vi "Render.vi"(8 "error in (no error)":errorcluster, 9 "IDrawable":refnum<class "IDrawable.lvclass">, 10 "2D Picture in":picture, 11 "2DPictureControl in":refnum<class "2DPictureControl.lvclass">) -> (0 "error out":errorcluster, 2 "2D Picture out":picture, 3 "2DPictureControl out":refnum<class "2DPictureControl.lvclass">)   [LabVIEW 2021, in "Picture2D.lvlib" / "2DPictureControl.lvclass"]
uses:
  2DPictureControl.lvclass
  IDrawable/IDrawable.lvclass
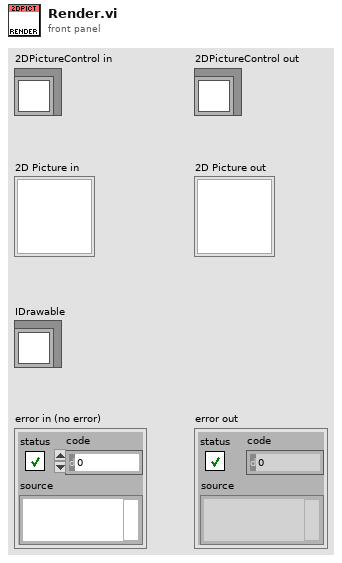
[diagram p1: front panel]
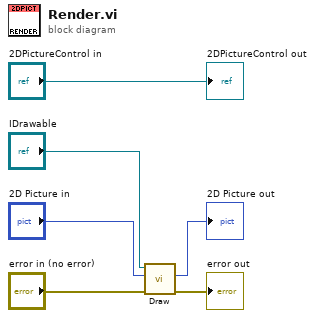
[diagram p0: block diagram]
diagram:
  n1 = call-dynamic "Draw.vi"("error in (no error)"="error in (no error)", "2D Picture in"="2D Picture in", "IDrawable in"="IDrawable") -> ("error out"=→"error out":errorcluster, "2D Picture out"=→"2D Picture out":picture)  [unwired: 6 in, 1 out]
  "2DPictureControl out" <- "2DPictureControl in"
